vi "Elevator_Globals.vi"() -> ()   [LabVIEW 2018]
uses:
  Subsytems/Elevator/Elevator_Notifier.ctl
  Subsytems/Elevator/Elevator_Control_Type.ctl
  Subsytems/Elevator/Elevator_Enum_States.ctl
panel:
  out "Up":bool
  out "Scoring":bool
  out "Elevator_Retracted":bool
  out "Elevator_Extended":bool
  out "Climb_Shifted":bool
  in  "Bottom_Elevator_Limit":string="Bottom_Elevator_Limit"
  in  "Top_Elevator_Limit":string="Top_Elevator_Limit"
  in  "Bottom_Climb_Limit_Front":string="Bottom_Climb_Limit_Front"
  in  "Top_Climb_Limit_Front":string="Top_Climb_Limit_Front"
  in  "Front_Brake":string="Front_Brake"
  in  "Elevator_Shift":string="Elevator_Shift"
  in  "Elevator_Slave":string="Elevator_Slave"
  in  "Elevator_Master":string="Elevator_Master"
  in  "Elevator_Execute_Notifier_Ref":refnum<notifier>
  in  "Elevator_Set_Notifier_Ref":refnum<notifier>
  in  "Elevator_Execute_Notifier":string="Elevator_Execute_Notifier"
  in  "Elevator_Set_Notifier":string="Elevator_Set_Notifier"
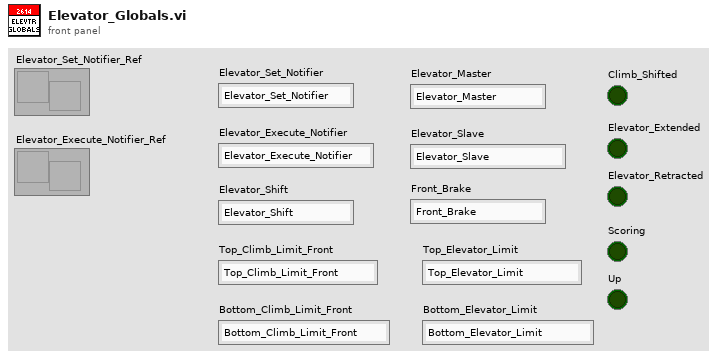
[diagram p1: front panel]
diagram:
